vi "rescale joystick.vi"(1 "postion (-1 to 1)":dbl, 2 "parameters":cluster{"max":dbl, "min":dbl, "center":dbl}) -> (0 "position (scaled)":dbl)   [LabVIEW 8.6]
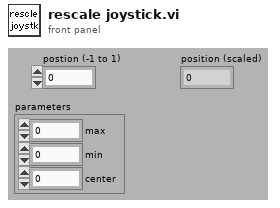
[diagram p1: front panel]
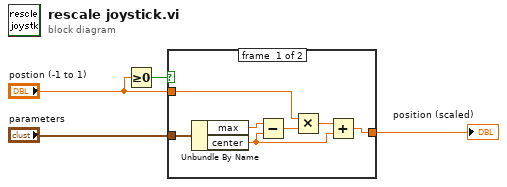
[diagram p0: block diagram]
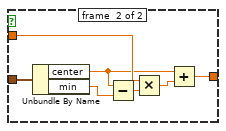
[diagram p2: hidden frame]
diagram:
  n1 = Greater Or Equal To 0?(x="postion (-1 to 1)") -> (x >= 0?=w4:bool)
  n2 = case shown="False" w4 {
    tunnel: "parameters" -> [w11 w18]
    tunnel: "postion (-1 to 1)" -> [w8 w16]
    tunnel: [w5 w13] -> w1
    frame #0 {
      n3 = Unbundle By Name(w11) -> ("max"=w10:dbl, "center"=w6:dbl)
      n4 = Subtract(x=w10, y=w6) -> (x-y=w9:dbl)
      n5 = Multiply(x=w8, y=w9) -> (x*y=w7:dbl)
      n6 = Add(x=w7, y=w6) -> (x+y=w5:dbl)
    }
    frame #1 {
      n7 = Unbundle By Name(w18) -> ("center"=w12:dbl, "min"=w14:dbl)
      n8 = Subtract(x=w12, y=w14) -> (x-y=w17:dbl)
      n9 = Multiply(x=w16, y=w17) -> (x*y=w15:dbl)
      n10 = Add(x=w12, y=w15) -> (x+y=w13:dbl)
    }
  }
  "position (scaled)" <- w1
